vi "Cafeluta.vi"() -> ()   [LabVIEW 2013]
panel:
  out "Ring":u16(ring)
  in  "Money":dbl=100.0 format="%#_13g"
  in  "10 cents":bool
  in  "20 cents":bool
  in  "50 cents":bool
  in  "5 euro":bool
  in  "2 euro":bool
  in  "1 euro":bool
  in  "HotWaterState":i32
  in  "Water temp.":i32
  in  "stop":bool
  in  "Mix % left":i32=100
  in  "Coffe button":bool
  out "Suggar MIx":dbl(slide) scale=0.0..100.0
  out "Coffe Mix":dbl(slide) scale=0.0..100.0
  out "Water temperature":dbl(knob) scale=0.0..120.0
  out "Water Level\n    Liters":dbl(slide) scale=0.0..30.0
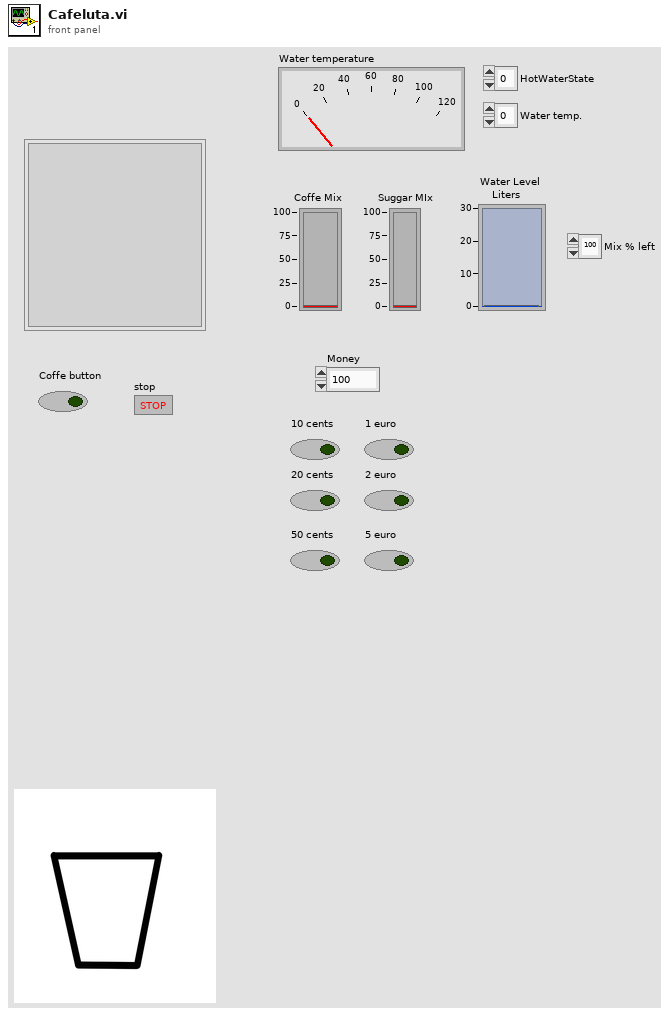
[diagram p1: front panel]
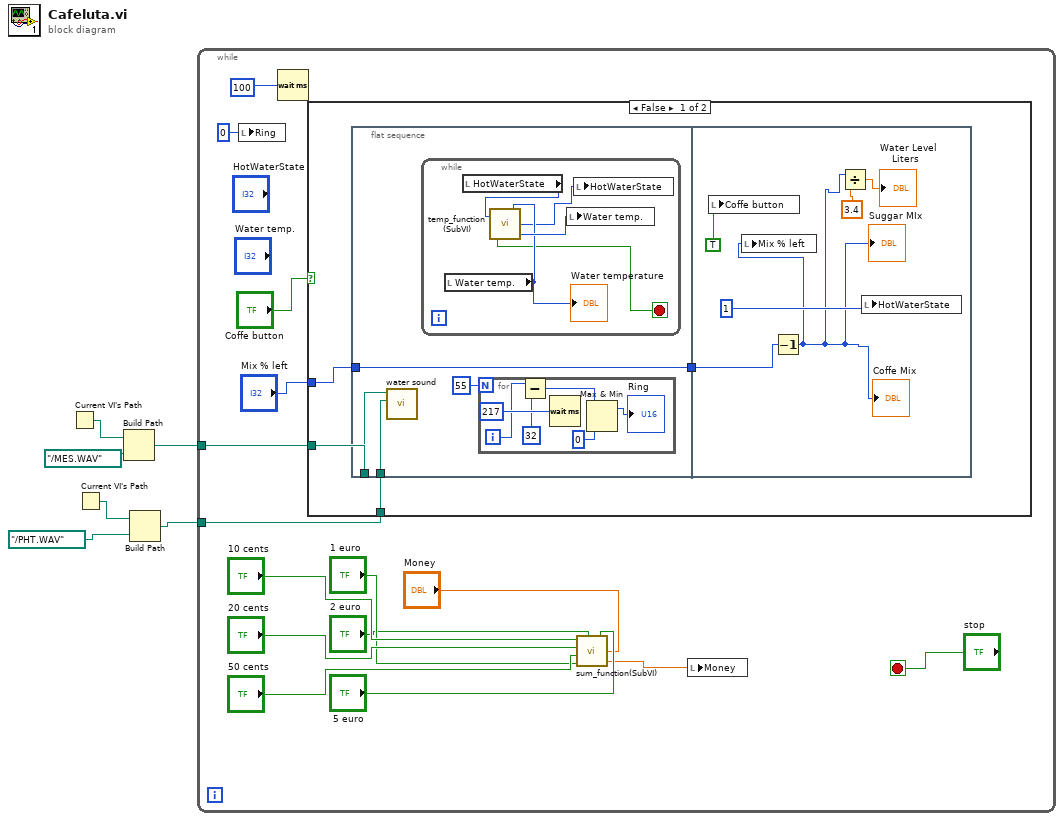
[diagram p0: block diagram]
diagram:
  n1 = Current VI's Path() -> (path=w6:path)
  n2 = Current VI's Path() -> (path=w5:path)
  n3 = Build Path(base path=w6, name or relative path=path "../MES.WAV") -> (appended path=w4:path)
  n4 = Build Path(base path=w5, name or relative path=path "../PHT.WAV") -> (appended path=w3:path)
  n5 = while {
    tunnel: w4 -> [w8]
    tunnel: w3 -> [w7]
    stop <- "stop" stop-if-true
    n6 = local write "Ring"(u16 0 ("Ring")) -> ()
    n7 = Wait (ms)(milliseconds to wait=100) -> ()  [unwired: 1 out]
    n8 = case shown="False" "Coffe button" {
      tunnel: "Mix % left" -> [w25 _]
      tunnel: w8 -> [w23 _]
      tunnel: w7 -> [w22 _]
      frame False {
        n9 = flat-sequence {
          tunnel: w25 -> [w27]
          tunnel: [w27] -> w24
          tunnel: w23 -> [w29]
          tunnel: w22 -> [w28]
          tunnel: w24 -> [w46]
          frame #0 {
            n10 = call "water sound.vi"("Path 2"=w28, "Path"=w29) -> ()  [unwired: 10 in]
            n11 = while {
              stop <- w36 stop-if-true
              n12 = local read "Water temp."() -> (w39:i32)
              "Water temperature" <- w39
              n13 = local read "HotWaterState"() -> (w38:i32)
              n14 = call "temp_function (SubVI).vi"("Water state IN"=w38, "Temp IN"=w39) -> ("Ready"=w36:bool, "Water state OUT"=w37:i32, "Temp OUT"=w40:i32)
              n15 = local write "Water temp."(w40) -> ()
              n16 = local write "HotWaterState"(w37) -> ()
            }
            n17 = for {
              N: 55 -> [_]
              i -> [w34]
              n18 = Subtract(x=w34, y=32) -> (x-y=w31:i32)
              n19 = Wait (ms)(milliseconds to wait=u32 217) -> ()  [unwired: 1 out]
              n20 = Max & Min(x=w31, y=0) -> (max(x,y)=→"Ring":i32)  [unwired: 1 out]
            }
          }
          frame #1 {
            n21 = local write "Coffe button"(TRUE) -> ()
            n22 = Decrement(x=w46) -> (x-1=w41:i32)
            "Suggar MIx" <- w41
            "Coffe Mix" <- w41
            n23 = local write "Mix % left"(w41) -> ()
            n24 = Divide(x=w41, y=3.4) -> (x/y=→"Water Level\n    Liters":dbl)
            n25 = local write "HotWaterState"(1) -> ()
          }
        }
      }
      frame True {
      }
    }
    n26 = call "sum_function(SubVI).vi"("10"="10 cents", "20"="20 cents", "50"="50 cents", "1"="1 euro", "2"="2 euro", "5"="5 euro", "Sum IN"="Money") -> ("Sum OUT"=w10:dbl)
    n27 = local write "Money"(w10) -> ()
  }
